vi "task 3 - backup.vi"() -> ()   [LabVIEW 2017]
uses:
  <vilib>/DAQmx/read.llb/DAQmx Read (Counter DBL 1Chan 1Samp).vi
  <vilib>/DAQmx/read.llb/DAQmx Read (Digital Bool 1Line 1Point).vi
  <vilib>/DAQmx/write.llb/DAQmx Write (Analog DBL 1Chan 1Samp).vi
  <vilib>/DAQmx/create/channels.llb/DAQmx Create Channel (AO-Voltage-Basic).vi
  <vilib>/DAQmx/create/channels.llb/DAQmx Create Channel (DI-Digital Input).vi
  <vilib>/DAQmx/create/channels.llb/DAQmx Create Channel (CI-Count Edges).vi
  <vilib>/DAQmx/miscellaneous.llb/DAQmx Fill In Error Info.vi
panel:
  in  "Numeric 2":dbl
  in  "Numeric":dbl
  in  "DAQmx Physical Channel 8":tag="Dev9/ao0"
  out "no of pulses 2":dbl format="%.2f"
  in  "DAQmx Physical Channel 7":tag="Dev9/ao0"
  out "no of pulses":dbl format="%.2f"
  out "Right":bool
  out "Bottom":bool
  out "Left":bool
  out "Top":bool
  in  "DAQmx Physical Channel 6":tag
  in  "DAQmx Physical Channel 5":tag
  in  "DAQmx Physical Channel 4":tag
  in  "DAQmx Physical Channel 3":tag
  in  "Motor stop":bool
  in  "DAQmx Physical Channel 2":tag="Dev9/ao0"
  in  "motor 2":dbl(slide)=3.2073478842720426 scale=-10.0..10.0
  in  "max Voltage":dbl
  in  "Min Voltage":dbl
  in  "DAQmx Physical Channel":tag="Dev9/ao0"
  in  "motor 1":dbl(slide)=3.2073478842720426 scale=-10.0..10.0
  in  "stop":bool
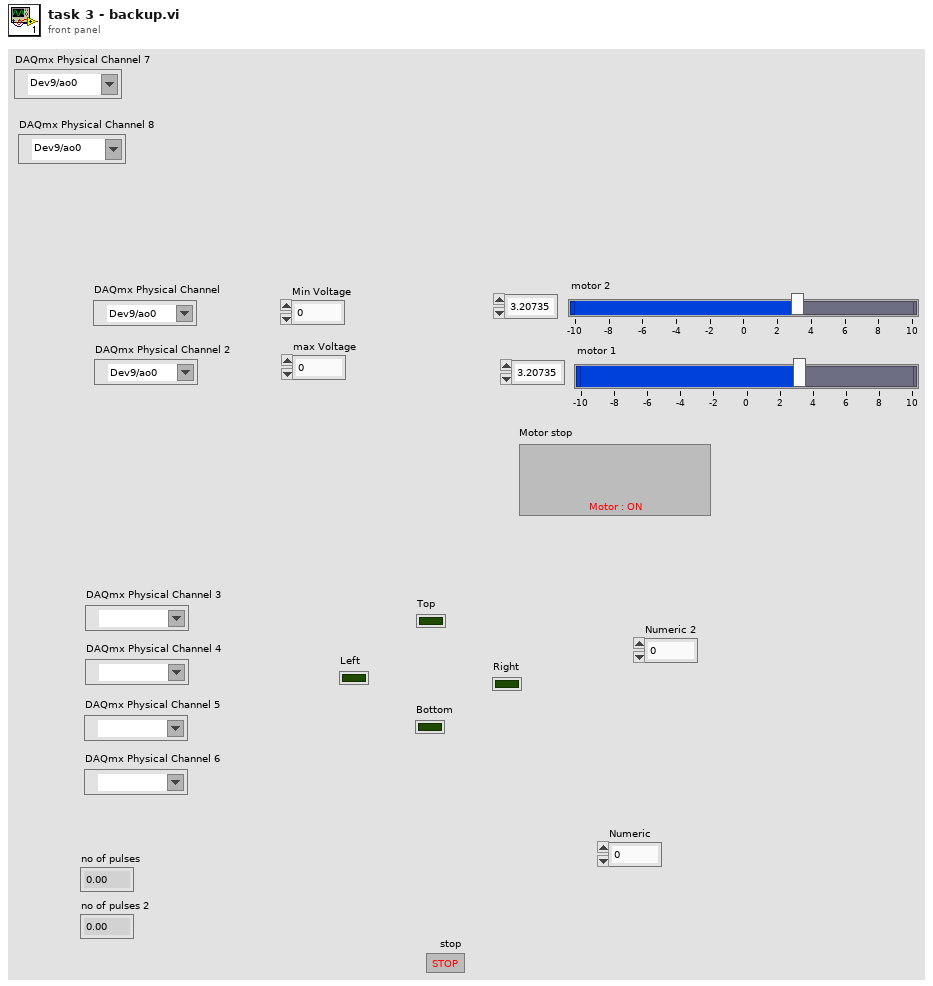
[diagram p1: front panel]
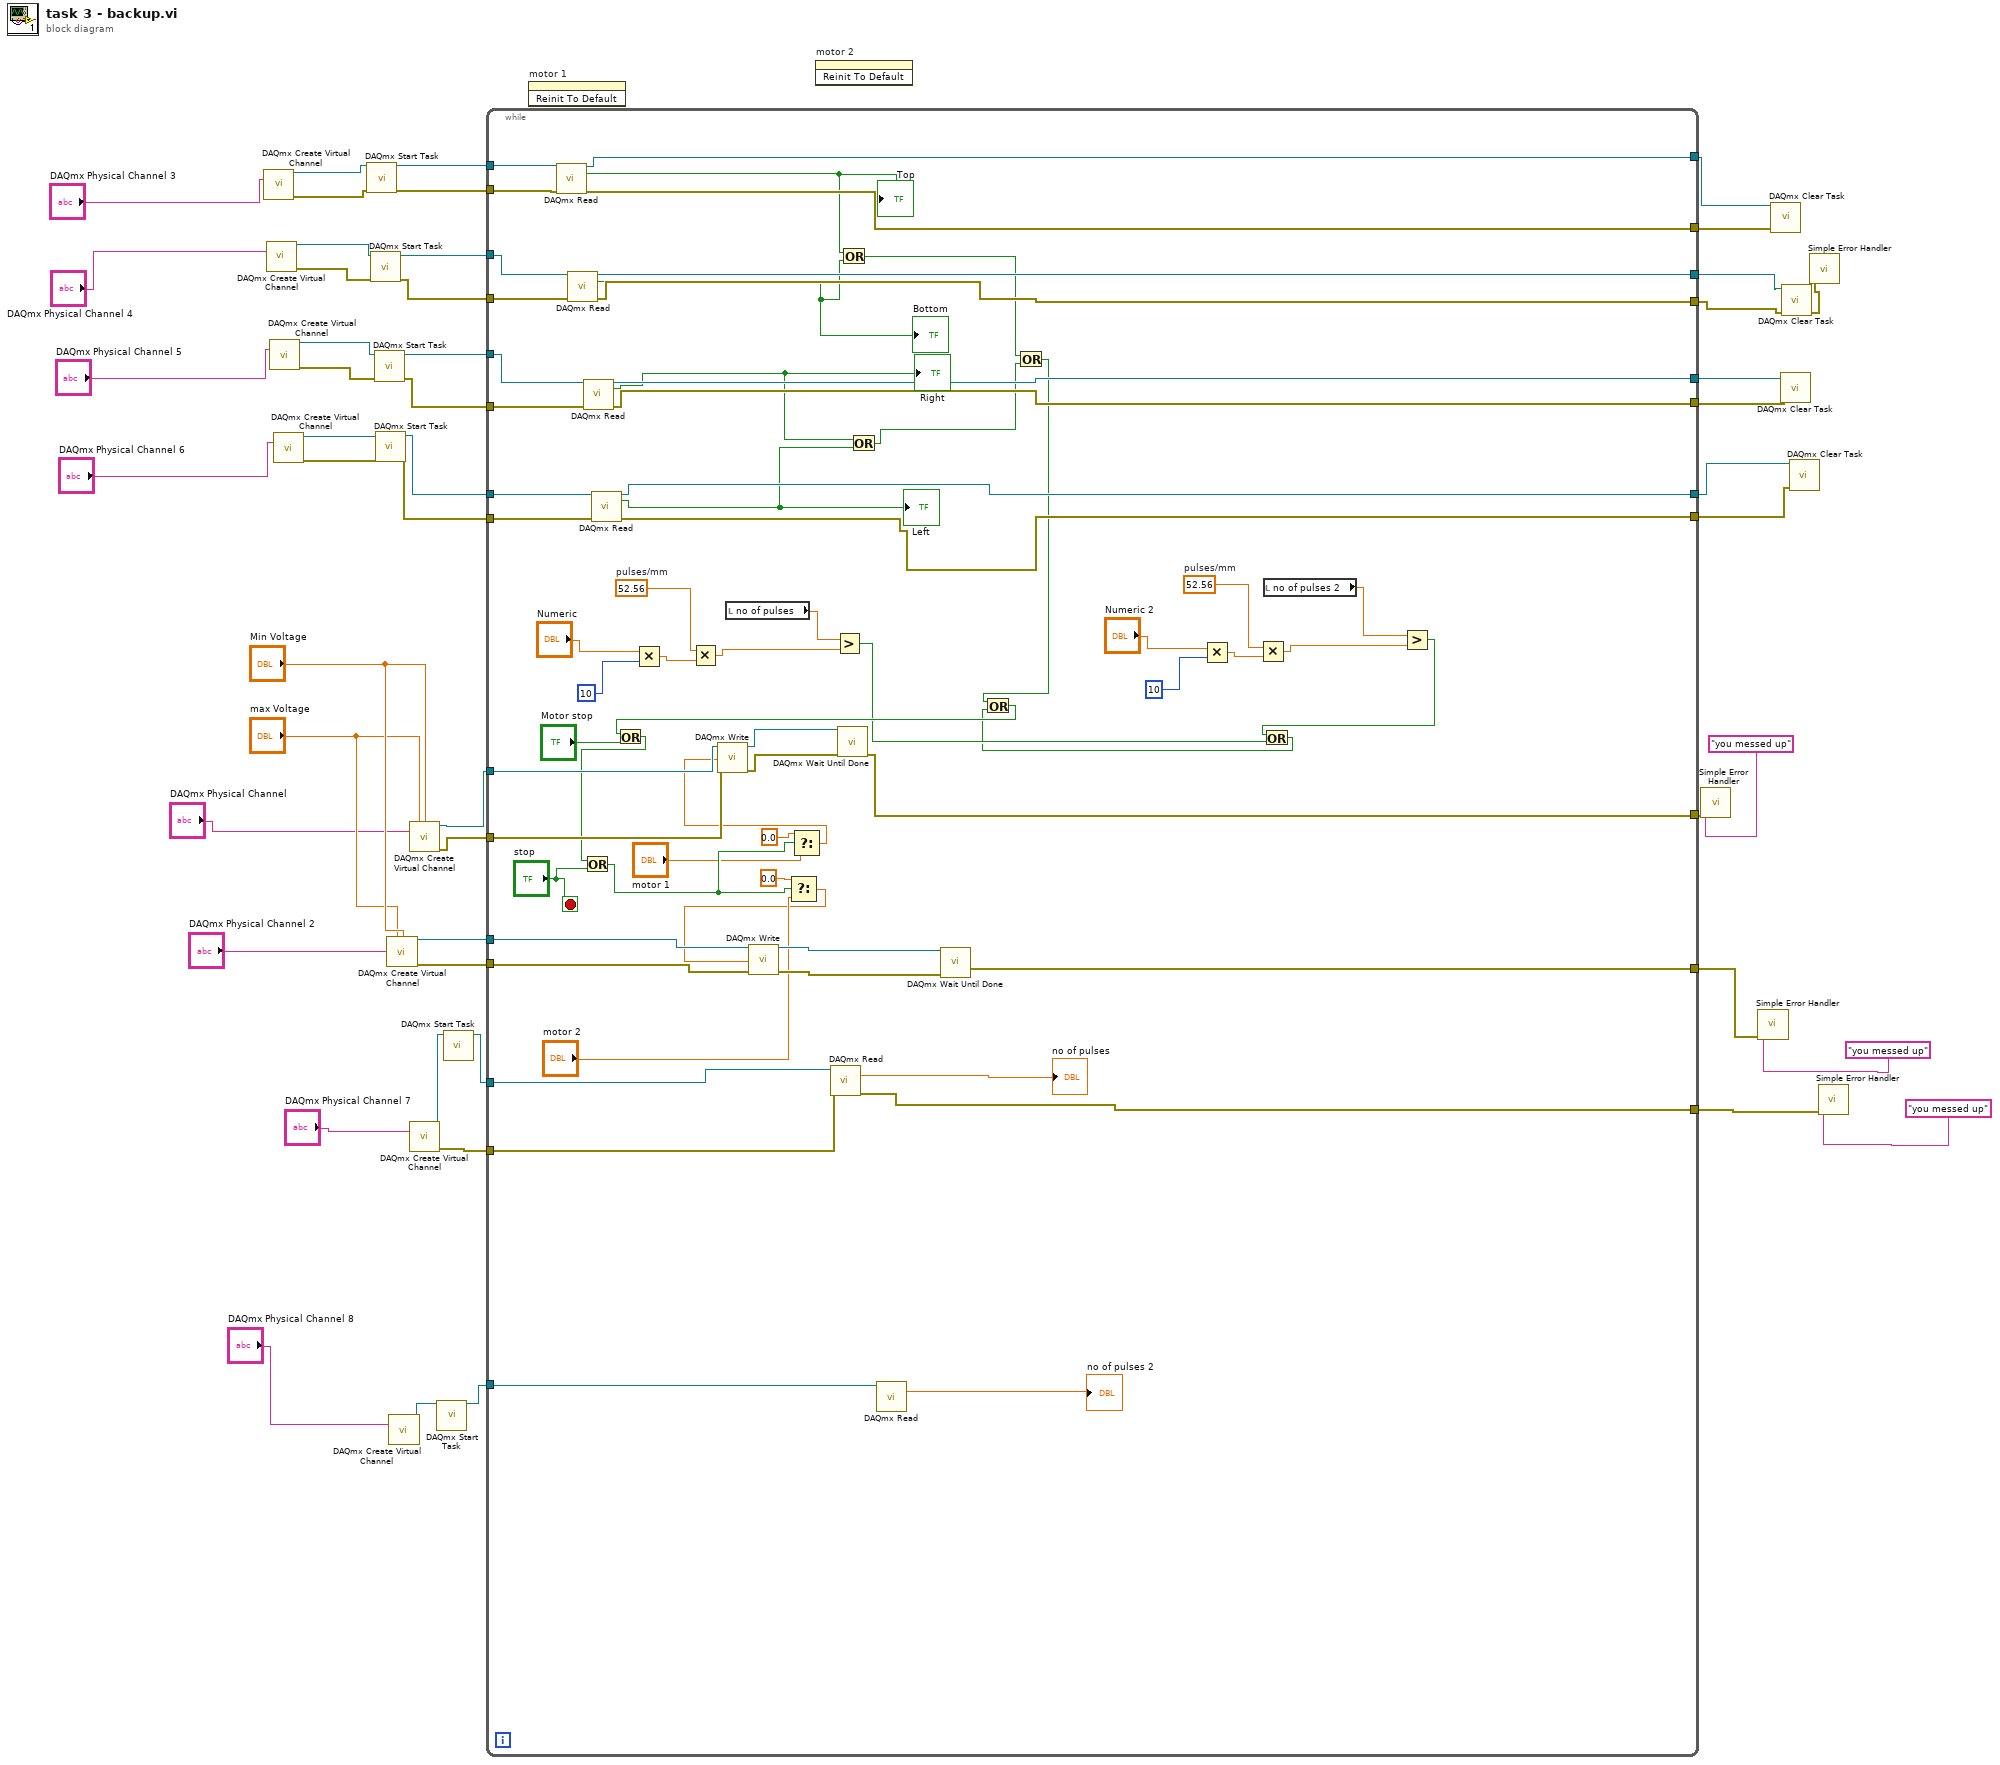
[diagram p0: block diagram]
diagram:
  n1 = call-poly <vilib>:"DAQmx Create Virtual Channel.vi"("lines"="DAQmx Physical Channel 3") -> ("task out"=w36:refnum<k21>, "error out"=w32:errorcluster)  [unwired: 13 in]
  n2 = call-poly <vilib>:"DAQmx Create Virtual Channel.vi"("lines"="DAQmx Physical Channel 4") -> ("task out"=w35:refnum<k21>, "error out"=w31:errorcluster)  [unwired: 13 in]
  n3 = call-poly <vilib>:"DAQmx Create Virtual Channel.vi"("lines"="DAQmx Physical Channel 5") -> ("task out"=w34:refnum<k21>, "error out"=w30:errorcluster)  [unwired: 13 in]
  n4 = call-poly <vilib>:"DAQmx Create Virtual Channel.vi"("lines"="DAQmx Physical Channel 6") -> ("task out"=w33:refnum<k21>, "error out"=w29:errorcluster)  [unwired: 13 in]
  n5 = call <vilib>:"DAQmx Start Task.vi"("task/channels in"=w36, "error in"=w32) -> ("task out"=w28:refnum<k21>, "error out"=w26:errorcluster)  [unwired: 12 in]
  n6 = call <vilib>:"DAQmx Start Task.vi"("task/channels in"=w35, "error in"=w31) -> ("task out"=w24:refnum<k21>, "error out"=w21:errorcluster)  [unwired: 12 in]
  n7 = call <vilib>:"DAQmx Start Task.vi"("task/channels in"=w34, "error in"=w30) -> ("task out"=w23:refnum<k21>, "error out"=w20:errorcluster)  [unwired: 12 in]
  n8 = call <vilib>:"DAQmx Start Task.vi"("task/channels in"=w33, "error in"=w29) -> ("task out"=w22:refnum<k21>, "error out"=w19:errorcluster)  [unwired: 12 in]
  n9 = call-poly <vilib>:"DAQmx Create Virtual Channel.vi"("maximum value"="max Voltage", "minimum value"="Min Voltage", "physical channels"="DAQmx Physical Channel 2") -> ("task out"=w46:refnum<k21>, "error out"=w42:errorcluster)  [unwired: 11 in]
  n10 = call-poly <vilib>:"DAQmx Create Virtual Channel.vi"("counter"="DAQmx Physical Channel 8") -> ("task out"=w4:refnum<k21>)  [unwired: 13 in, 1 out]
  n11 = call-poly <vilib>:"DAQmx Create Virtual Channel.vi"("maximum value"="max Voltage", "minimum value"="Min Voltage", "physical channels"="DAQmx Physical Channel") -> ("task out"=w49:refnum<k21>, "error out"=w41:errorcluster)  [unwired: 11 in]
  n12 = call-poly <vilib>:"DAQmx Create Virtual Channel.vi"("counter"="DAQmx Physical Channel 7") -> ("task out"=w6:refnum<k21>, "error out"=w7:errorcluster)  [unwired: 13 in]
  n13 = call <vilib>:"DAQmx Start Task.vi"("task/channels in"=w4) -> ("task out"=w3:refnum<k21>)  [unwired: 13 in, 1 out]
  n14 = call <vilib>:"DAQmx Start Task.vi"("task/channels in"=w6) -> ("task out"=w5:refnum<k21>)  [unwired: 13 in, 1 out]
  n15 = while {
    tunnel: w49 -> [w115]
    tunnel: [w112] -> w48
    tunnel: w46 -> [w109]
    tunnel: [w108] -> w45
    tunnel: w42 -> [w106]
    tunnel: w41 -> [w105]
    tunnel: w28 -> [w97]
    tunnel: [w96] -> w27
    tunnel: w26 -> [w95]
    tunnel: [w94] -> w25
    tunnel: w24 -> [w93]
    tunnel: w23 -> [w92]
    tunnel: w22 -> [w91]
    tunnel: w21 -> [w90]
    tunnel: w20 -> [w89]
    tunnel: w19 -> [w88]
    tunnel: [w87] -> w18
    tunnel: [w86] -> w17
    tunnel: [w85] -> w16
    tunnel: [w84] -> w15
    tunnel: [w83] -> w14
    tunnel: [w82] -> w13
    tunnel: [w81] -> w10
    tunnel: w5 -> [w80]
    tunnel: w7 -> [w79]
    tunnel: w3 -> [w68]
    stop <- "stop" stop-if-true
    w55 = 52.56  # pulses/mm
    w63 = 52.56  # pulses/mm
    n16 = call-poly <vilib>:"DAQmx Read.vi"("task/channels in"=w97, "error in"=w95) -> ("task out"=w96:refnum<k21>, "data"=w77:bool, "error out"=w94:errorcluster)  [unwired: 11 in]
    "Top" <- w77
    n17 = call-poly <vilib>:"DAQmx Read.vi"("task/channels in"=w93, "error in"=w90) -> ("task out"=w87:refnum<k21>, "data"=w76:bool, "error out"=w84:errorcluster)  [unwired: 11 in]
    "Bottom" <- w76
    n18 = call-poly <vilib>:"DAQmx Read.vi"("task/channels in"=w92, "error in"=w89) -> ("task out"=w86:refnum<k21>, "data"=w74:bool, "error out"=w83:errorcluster)  [unwired: 11 in]
    "Right" <- w74
    n19 = call-poly <vilib>:"DAQmx Read.vi"("task/channels in"=w91, "error in"=w88) -> ("task out"=w85:refnum<k21>, "data"=w73:bool, "error out"=w82:errorcluster)  [unwired: 11 in]
    "Left" <- w73
    n20 = Multiply(x="Numeric", y=10) -> (x*y=w62:dbl)
    n21 = Multiply(x=w63, y=w62) -> (x*y=w61:dbl)
    n22 = local read "no of pulses"() -> (w60:dbl)
    n23 = call-poly <vilib>:"DAQmx Read.vi"("task/channels in"=w80, "error in"=w79) -> ("data"=→"no of pulses":dbl, "error out"=w81:errorcluster)  [unwired: 11 in, 1 out]
    n24 = Greater?(x=w60, y=w61) -> (0:w53:bool)
    n25 = Or(x=w77, y=w76) -> (x .or. y?=w75:bool)
    n26 = Or(x=w74, y=w73) -> (x .or. y?=w72:bool)
    n27 = call-poly <vilib>:"DAQmx Read.vi"("task/channels in"=w68) -> ("data"=→"no of pulses 2":dbl)  [unwired: 12 in, 2 out]
    n28 = Or(x=w75, y=w72) -> (x .or. y?=w67:bool)
    n29 = Multiply(x="Numeric 2", y=10) -> (x*y=w58:dbl)
    n30 = Multiply(x=w55, y=w58) -> (x*y=w59:dbl)
    n31 = local read "no of pulses 2"() -> (w51:dbl)
    n32 = Greater?(x=w51, y=w59) -> (0:w54:bool)
    n33 = Or(x=w54, y=w53) -> (x .or. y?=w52:bool)
    n34 = Or(x=w67, y=w52) -> (x .or. y?=w66:bool)
    n35 = Or(x=w66, y="Motor stop") -> (x .or. y?=w70:bool)
    n36 = Or(x=w70, y="stop") -> (x .or. y?=w102:bool)
    n37 = Select(t=0.0, s=w102, f="motor 2") -> (s? t:f=w98:dbl)
    n38 = call-poly <vilib>:"DAQmx Write.vi"("task/channels in"=w109, "data"=w98, "error in"=w106) -> ("task out"=w110:refnum<k21>, "error out"=w111:errorcluster)  [unwired: 10 in, 1 out]
    n39 = Select(t=0.0 ("s? t:f"), s=w102, f="motor 1") -> (s? t:f=w99:dbl)
    n40 = call-poly <vilib>:"DAQmx Write.vi"("task/channels in"=w115, "data"=w99, "error in"=w105) -> ("task out"=w114:refnum<k21>, "error out"=w113:errorcluster)  [unwired: 10 in, 1 out]
    n41 = call <vilib>:"DAQmx Wait Until Done.vi"("task/channels in"=w114, "error in"=w113) -> ("error out"=w112:errorcluster)  [unwired: 12 in, 1 out]
    n42 = call <vilib>:"DAQmx Wait Until Done.vi"("task/channels in"=w110, "error in"=w111) -> ("error out"=w108:errorcluster)  [unwired: 12 in, 1 out]
  }
  n43 = invoke on="motor 1" class="Slide (strict)" method="Reinit To Default"() -> ()  [unwired: 3 in, 3 out]
  n44 = invoke on="motor 2" class="Slide (strict)" method="Reinit To Default"() -> ()  [unwired: 3 in, 3 out]
  n45 = call <vilib>:"Simple Error Handler.vi"("error source (\" \")"="you messed up" ("error source (\" \")"), "error in (no error)"=w48) -> ()  [unwired: 3 in, 5 out]
  n46 = call <vilib>:"Simple Error Handler.vi"("error source (\" \")"="you messed up" ("error source (\" \")"), "error in (no error)"=w45) -> ()  [unwired: 3 in, 5 out]
  n47 = call <vilib>:"DAQmx Clear Task.vi"("task in"=w27, "error in"=w25) -> ()  [unwired: 13 in, 1 out]
  n48 = call <vilib>:"DAQmx Clear Task.vi"("task in"=w17, "error in"=w14) -> ()  [unwired: 13 in, 1 out]
  n49 = call <vilib>:"DAQmx Clear Task.vi"("task in"=w18, "error in"=w15) -> ("error out"=w12:errorcluster)  [unwired: 13 in]
  n50 = call <vilib>:"DAQmx Clear Task.vi"("task in"=w16, "error in"=w13) -> ()  [unwired: 13 in, 1 out]
  n51 = call <vilib>:"Simple Error Handler.vi"("error in (no error)"=w12) -> ()  [unwired: 4 in, 5 out]
  n52 = call <vilib>:"Simple Error Handler.vi"("error source (\" \")"="you messed up" ("error source (\" \")"), "error in (no error)"=w10) -> ()  [unwired: 3 in, 5 out]
